vi "Expotec.vi"() -> ()   [LabVIEW 2013]
uses:
  <vilib>/Instr/_visa.llb/VISA Configure Serial Port (Instr).vi
panel:
  in  "Bomba VEntiladores":bool
  in  "VEntiladores 1-2":bool
  in  "VEntilador 1":bool
  in  "Bomba":bool
  out "Lectura Temperatura\nAmbiente":dbl(knob) scale=0.0..100.0
  out "Lectura Humedad":dbl(knob) scale=0.0..100.0
  in  "stop":bool
  out "String":string
  in  "VISA resource name":refnum<visa-resource-name>
  out "Temperatura Analogica":dbl(knob) scale=0.0..50.0
  out "Lectura en tierra":dbl(knob) scale=0.0..1024.0
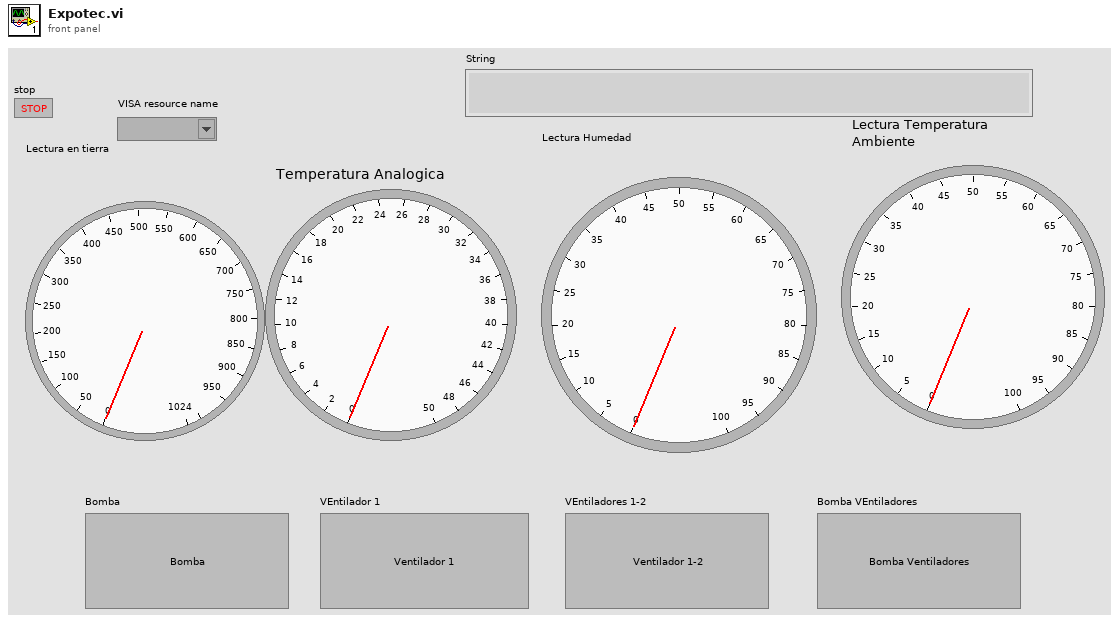
[diagram p1: front panel]
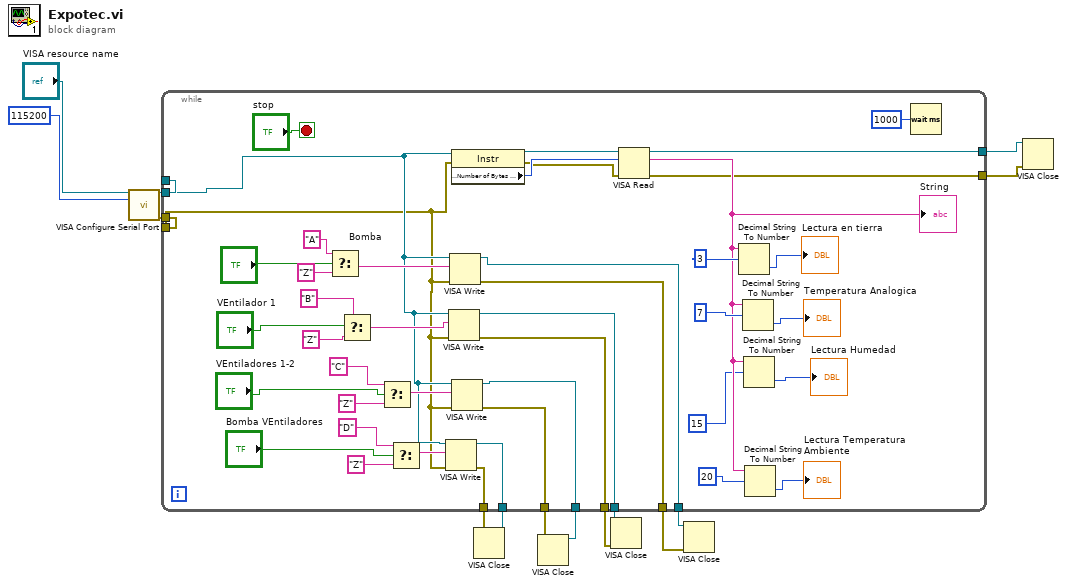
[diagram p0: block diagram]
diagram:
  n1 = call-poly "VISA Configure Serial Port"("VISA resource name"="VISA resource name", "baud rate (9600)"=u32 115200) -> ("VISA resource name out"=w11:refnum<visa-resource-name>, "error out"=w12:errorcluster)  [unwired: 12 in]
  n2 = while {
    tunnel: w12 -> [_]
    tunnel: w11 -> [_]
    tunnel: w12 -> [w19]
    tunnel: w11 -> [w20]
    tunnel: [w31] -> w10
    tunnel: [w30] -> w9
    tunnel: [w29] -> w8
    tunnel: [w28] -> w7
    tunnel: [w27] -> w6
    tunnel: [w26] -> w5
    tunnel: [w25] -> w4
    tunnel: [w24] -> w3
    tunnel: [w22] -> w2
    tunnel: [w21] -> w1
    stop <- "stop" stop-if-true
    n3 = Select(t="A", s="Bomba", f="Z") -> (s? t:f=w34:string)
    n4 = Select(t="B", s="VEntilador 1", f="Z") -> (s? t:f=w35:string)
    n5 = Select(t="C", s="VEntiladores 1-2", f="Z") -> (s? t:f=w33:string)
    n6 = Select(t="D", s="Bomba VEntiladores", f="Z") -> (s? t:f=w32:string)
    n7 = VISA Write(VISA resource name=w20, write buffer=w32, error in (no error)=w19) -> (VISA resource name out=w29:refnum<visa-resource-name>, error out=w28:errorcluster)  [unwired: 1 out]
    n8 = VISA Write(VISA resource name=w20, write buffer=w35, error in (no error)=w19) -> (VISA resource name out=w26:refnum<visa-resource-name>, error out=w27:errorcluster)  [unwired: 1 out]
    n9 = VISA Write(VISA resource name=w20, write buffer=w34, error in (no error)=w19) -> (VISA resource name out=w25:refnum<visa-resource-name>, error out=w24:errorcluster)  [unwired: 1 out]
    n10 = property class="Instr"(reference=w20, error in=w19) -> (reference out=w17:refnum<visa-resource-name>, error out=w16:errorcluster, "Serial Settings:Number of Bytes at Serial Port"=w18:u32)
    n11 = VISA Write(VISA resource name=w20, write buffer=w33, error in (no error)=w19) -> (VISA resource name out=w31:refnum<visa-resource-name>, error out=w30:errorcluster)  [unwired: 1 out]
    n12 = VISA Read(VISA resource name=w17, byte count=w18, error in (no error)=w16) -> (VISA resource name out=w22:refnum<visa-resource-name>, read buffer=w54:string, error out=w21:errorcluster)  [unwired: 1 out]
    "String" <- w54
    n13 = Decimal String To Number(string=w54, offset=3) -> (number=→"Lectura en tierra":i32)  [unwired: 1 in, 1 out]
    n14 = Decimal String To Number(string=w54, offset=7) -> (number=→"Temperatura Analogica":i32)  [unwired: 1 in, 1 out]
    n15 = Decimal String To Number(string=w54, offset=15) -> (number=→"Lectura Humedad":i32)  [unwired: 1 in, 1 out]
    n16 = Decimal String To Number(string=w54, offset=20) -> (number=→"Lectura Temperatura\nAmbiente":i32)  [unwired: 1 in, 1 out]
    n17 = Wait (ms)(milliseconds to wait=u32 1000) -> ()  [unwired: 1 out]
  }
  n18 = VISA Close(VISA resource name=w8, error in (no error)=w7) -> ()  [unwired: 1 out]
  n19 = VISA Close(VISA resource name=w10, error in (no error)=w9) -> ()  [unwired: 1 out]
  n20 = VISA Close(VISA resource name=w5, error in (no error)=w6) -> ()  [unwired: 1 out]
  n21 = VISA Close(VISA resource name=w4, error in (no error)=w3) -> ()  [unwired: 1 out]
  n22 = VISA Close(VISA resource name=w2, error in (no error)=w1) -> ()  [unwired: 1 out]
